vi "Unpain Button.vi"(8 "error in (no error)":errorcluster, 10 "Old Button":i32, 11 "Button States in":refnum<class "Button.lvclass">[](array[class])) -> (0 "error out":errorcluster, 3 "Button States out":refnum<class "Button.lvclass">[](array[class]))   [LabVIEW 2012, in "Toolbar.xctl"]
doc: "Unpaints a button when the cursor moves out"
uses:
  Toolbar.xctl
  Button_Class/Button.lvclass
  Button_Class/Type Defs/Button Status.ctl
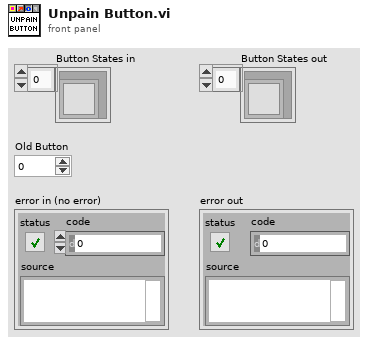
[diagram p1: front panel]
types:
  T1 = typedef "Button.lvclass/Button Status.ctl" = enum16{"Off", "Hover", "On", "Disabled"}
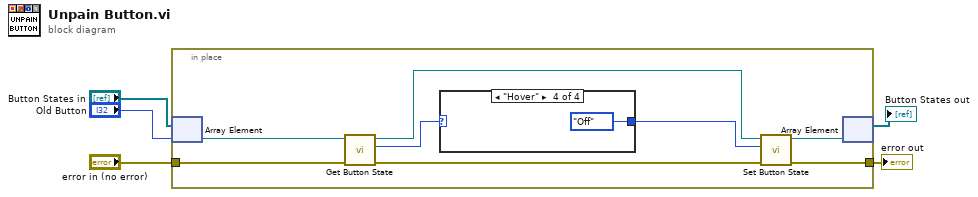
[diagram p0: block diagram]
diagram:
  n1 = in-place {
    in-place-border: "error in (no error)" -> [w9]
    in-place-border: [w6] -> w5
    n2 = in-place-array #1("Button States in", "Old Button") -> (w13:refnum<class "Button.lvclass">)
    n3 = call-dynamic "Get Button State.vi"("error in (no error)"=w9, "Button in"=w13) -> ("error out"=w8:errorcluster, "State"=w11:T1, "Button out"=w12:refnum<class "Button.lvclass">)  [unwired: 1 in, 6 out]
    n4 = case shown="\"Hover\"" w11 {
      selector: w11 -> [w14 w15 w16 _]
      tunnel: [w14 w15 w16 Button_Status."Off" ("State")] -> w10
      frame "Off", Default {
      }
      frame "On" {
      }
      frame "Disabled" {
      }
      frame "Hover" {
      }
    }
    n5 = call-dynamic "Set Button State.vi"("error in (no error)"=w8, "State"=w10, "Button in"=w12) -> ("error out"=w6:errorcluster, "Button out"=w7:refnum<class "Button.lvclass">)  [unwired: 7 out]
    n6 = in-place-array #1(w7) -> (→"Button States out":refnum<class "Button.lvclass">[])  [unwired: 1 out]
  }
  "error out" <- w5
